vi "Login and Get.vi"() -> ()   [LabVIEW 2019]
uses:
  firebase.lvclass
panel:
  out "Json String":string
  in  "endPoint":string
  out "firebase out":refnum<class "firebase.lvclass">
  in  "Email":string
  in  "Password":string
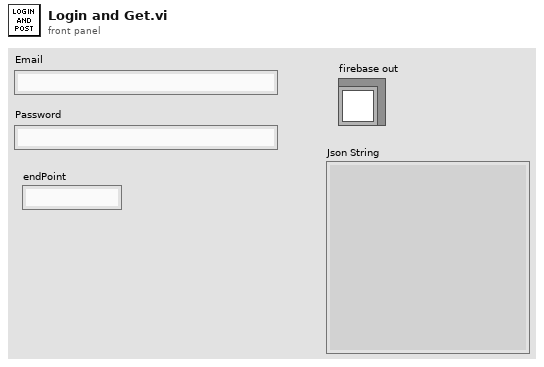
[diagram p1: front panel]
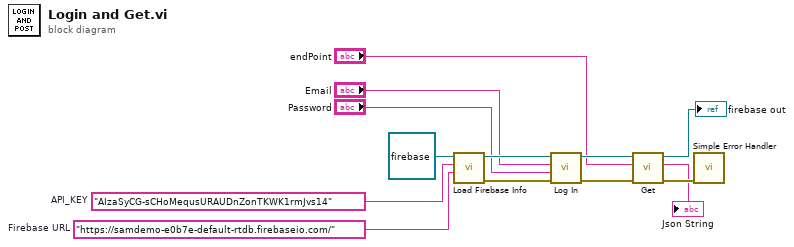
[diagram p0: block diagram]
diagram:
  w7 = "AIzaSyCG-sCHoMequsURAUDnZonTKWK1rmJvs14"  # API_KEY
  w8 = "https://samdemo-e0b7e-default-rtdb.firebaseio.com/"  # Firebase URL
  n1 = call "Load Firebase Info.vi"("Firebase URL"=w8, "API_KEY"=w7, "firebase in"=refnum<class "firebase.lvclass"> refnum ("firebase.lvclass")) -> ("error out"=w13:errorcluster, "firebase out"=w11:refnum<class "firebase.lvclass">)  [unwired: 7 in]
  n2 = call-dynamic "Log In.vi"("error in"=w13, "password"="Password", "email"="Email", "firebase in"=w11) -> ("error out"=w5:errorcluster, "firebase out"=w6:refnum<class "firebase.lvclass">)  [unwired: 6 in]
  n3 = call-dynamic "Get.vi"("error in"=w5, "endPoint"="endPoint", "firebase in"=w6) -> ("error out"=w4:errorcluster, "Json String"=→"Json String":string, "firebase out"=→"firebase out":refnum<class "firebase.lvclass">)  [unwired: 6 in]
  n4 = call <vilib>:"Simple Error Handler.vi"("error in (no error)"=w4) -> ()  [unwired: 4 in, 5 out]
